vi "AttrGetIsConnected.vi"(8 "error in":errorcluster, 11 "CanHandleIn":T1) -> (0 "error out":errorcluster, 2 "State":bool, 3 "CanHandleOut":T1)   [LabVIEW 2011, in "Konvolucio MCAN120803.lvlib"]
uses:
  <instrlib>/Konvolucio MCAN120803/Konvolucio MCAN120803.lvlib
  <instrlib>/Konvolucio MCAN120803/Types/CanHandleType.ctl
  C:/Program Files/National Instruments/LabVIEW 2011/instr.lib/Konvolucio MCAN120803/Private/Konvolucio.MCAN120803.API.dll
  Private/Konvolucio.MCAN120803.API.dll
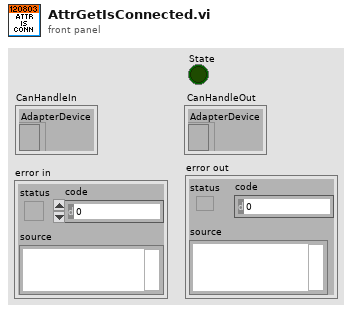
[diagram p1: front panel]
types:
  T1 = typedef "Konvolucio MCAN120803.lvlib/CanHandleType.ctl" = cluster{"AdapterDevice":refnum<k24>}
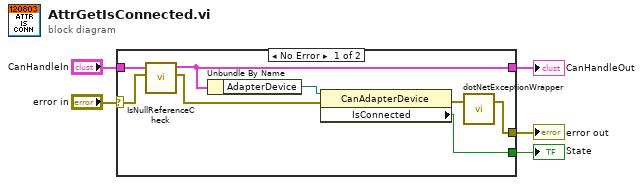
[diagram p0: block diagram]
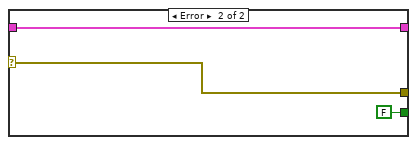
[diagram p2: hidden frame]
diagram:
  n1 = case shown="No Error" "error in" {
    selector: "error in" -> [w6 w16]
    tunnel: [w10 w16] -> w5
    tunnel: [w13 FALSE ("IsOpen")] -> w3
    tunnel: [w8 w14] -> w1
    tunnel: "CanHandleIn" -> [w9 w14]
    frame No Error {
      n2 = call <instrlib>:"IsNullReferenceCheck.vi"("error in"=w6, "MCanHandleIn"=w9) -> ("error out"=w7:errorcluster, "MCanHandleOut"=w8:T1)  [unwired: 5 in]
      n3 = Unbundle By Name(w8) -> ("AdapterDevice"=w12:refnum<k24>)
      n4 = property class="CanAdapterDevice"(reference=w12, error in=w7) -> (error out=w11:errorcluster, "IsConnected"=w13:bool)  [unwired: 1 out]
      n5 = call <instrlib>:"dotNetExceptionWrapper.vi"("error in"=w11) -> ("error out"=w10:errorcluster)  [unwired: 2 in]
    }
    frame Error {
    }
  }
  "error out" <- w5
  "CanHandleOut" <- w1
  "State" <- w3
